vi "Outputs.vi"(8 "error in (no error)":errorcluster, 11 "State in":T1={"State"=enum."Idle", "Start Time"=timestamp(0 s since 1904-01-01), "Configuration"={"Cycle Period"=0.0, "Setpoint Entry"=0.0, "Output Device"=enum."Huber Ministat 230", "Huber Ministat 230 Settings"={"VISA resource name"="", "Simulated?"=FALSE}, "Lauda Settings"={"VISA resource name"="", "Simulated?"=FALSE, "Pump Power"=2}, "Julabo FP-50 Settings"={"VISA resource name"="", "Simulated?"=FALSE, "Pump Power"=2}, "Internal Control?"=FALSE, "Huber Unistat 410 Settings"={"VISA resource name"="", "Address"=0, "Simulated?"=FALSE}}, "Current Time"=timestamp(0 s since 1904-01-01), "First Iteration"=FALSE, "Data"={"TCU Speed"=0.0, "Temperature"=0.0}, "Process Name"="", "TCU On?"=FALSE, "Output Error"=FALSE, "Start Log"=FALSE, "Power Level Changed"=FALSE} {"Configuration"."Huber Unistat 410 Settings"."Address" min=0 max=99 format="%02.0f"; "Configuration"."Julabo FP-50 Settings"."Pump Power" min=0 max=8 step=1; "Configuration"."Lauda Settings"."Pump Power" min=0 max=8 step=1}) -> (0 "error out":errorcluster, 3 "State out":T1={"State"=enum."Idle", "Start Time"=timestamp(0 s since 1904-01-01), "Configuration"={"Cycle Period"=0.0, "Setpoint Entry"=0.0, "Output Device"=enum."Huber Ministat 230", "Huber Ministat 230 Settings"={"VISA resource name"="", "Simulated?"=FALSE}, "Lauda Settings"={"VISA resource name"="", "Simulated?"=FALSE, "Pump Power"=2}, "Julabo FP-50 Settings"={"VISA resource name"="", "Simulated?"=FALSE, "Pump Power"=2}, "Internal Control?"=FALSE, "Huber Unistat 410 Settings"={"VISA resource name"="", "Address"=0, "Simulated?"=FALSE}}, "Current Time"=timestamp(0 s since 1904-01-01), "First Iteration"=FALSE, "Data"={"TCU Speed"=0.0, "Temperature"=0.0}, "Process Name"="", "TCU On?"=FALSE, "Output Error"=FALSE, "Start Log"=FALSE, "Power Level Changed"=FALSE} {"Configuration"."Huber Unistat 410 Settings"."Address" min=0 max=99 format="%02.0f"; "Configuration"."Julabo FP-50 Settings"."Pump Power" min=0 max=8 step=1; "Configuration"."Lauda Settings"."Pump Power" min=0 max=8 step=1})   [LabVIEW 2018, in "TCU Module.lvlib" / "TCU Module Engine.lvlib"]
uses:
  TCU Module Engine.lvlib
  TCU State Cluster.ctl
  State Enum.ctl
  TCU Module Settings Cluster.ctl
  Output Devices.ctl
  Huber TCU/Huber Settings.ctl
  Lauda Integral XT-150 TCU/Lauda Settings.ctl
  Julabo Type 1 TCU/Julabo Type 1 TCU Folder/Julabo FP-50 Settings.ctl
  Huber Unistat 410 TCU/Huber Unistat 410 RS485 Settings.ctl
  Tag VIs/Tag FGV Operation Enum.ctl
  Shared Variables/Dynamic Shared Variables.lvlib
  Huber TCU/Huber Ministat 230 TCU.lvlib
  Lauda Integral XT-150 TCU/Lauda TCU.lvlib
  Julabo Type 1 TCU/Julabo Type 1 TCU Folder/Julabo Type FP-50 TCU.lvlib
  Huber Unistat 410 TCU/Huber Unistat 410 TCU.lvlib
  TCU Module.lvlib
panel:
  # "Output Instruments"
  # "Output Instruments"
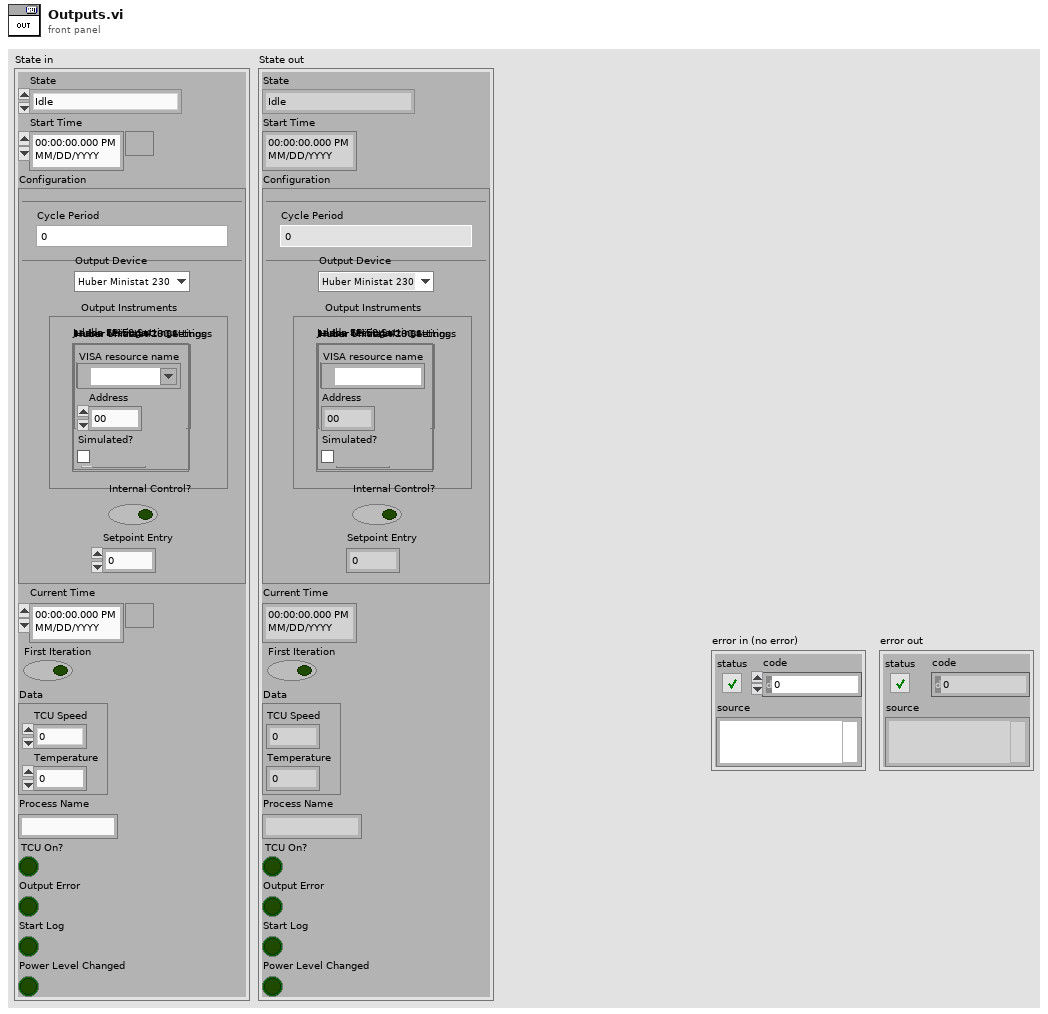
[diagram p1: front panel]
types:
  T1 = typedef "TCU Module.lvlib/TCU Module Engine.lvlib/TCU State Cluster.ctl" = cluster{"State":T2, "Start Time":timestamp, "Configuration":T3, "Current Time":timestamp, "First Iteration":bool, "Data":cluster{"TCU Speed":dbl, "Temperature":dbl}, "Process Name":string, "TCU On?":bool, "Output Error":bool, "Start Log":bool, "Power Level Changed":bool}
  T2 = typedef "TCU Module.lvlib/TCU Module Engine.lvlib/State Enum.ctl" = enum16{"Measuring", "Idle", "Paused"}
  T3 = typedef "TCU Module.lvlib/TCU Module Settings Cluster.ctl" = cluster{"Cycle Period":dbl, "Setpoint Entry":dbl, "Output Device":T4, "Huber Ministat 230 Settings":T5, "Lauda Settings":T6, "Julabo FP-50 Settings":T7, "Internal Control?":bool, "Huber Unistat 410 Settings":T8}
  T4 = typedef "Output Devices.ctl" = enum16{"Default", "Huber Ministat 230", "Huber Unistat 410", "Lauda XT-150", "Julabo FP-50"}
  T5 = typedef "Huber Ministat 230 TCU.lvlib/Huber Settings.ctl" = cluster{"VISA resource name":refnum<visa-resource-name>, "Simulated?":bool}
  T6 = typedef "Lauda TCU.lvlib/Lauda Settings.ctl" = cluster{"VISA resource name":refnum<visa-resource-name>, "Simulated?":bool, "Pump Power":i32}
  T7 = typedef "Julabo Type FP-50 TCU.lvlib/Julabo FP-50 Settings.ctl" = cluster{"VISA resource name":refnum<visa-resource-name>, "Simulated?":bool, "Pump Power":i32}
  T8 = typedef "Huber Unistat 410 TCU.lvlib/Huber Unistat 410 RS485 Settings.ctl" = cluster{"VISA resource name":refnum<visa-resource-name>, "Address":i8, "Simulated?":bool}
  T9 = typedef "Tag FGV Operation Enum.ctl" = enum16{"Init", "Set Notification Queue", "Create Tag", "Commit", "Write Tag (Numeric)", "Write Tag (Boolean)", "Read All Tags", "Read One Tag", "Delete Tag Category", "Set Alarm Parameters (Numeric)", "Set Alarm Parameters (Boolean)", "Enable All Alarms", "Disable All Alarms", "Delete All Tags", "Read Alarms", "Ack Alarm", "Read Alarm Parameters (Numeric)", "Read Alarm Parameters (Boolean)"}
  T10 = typedef "TCU Module.lvlib/TCU Module Tag Names Cluster.ctl" = cluster{"TCU Temp":string, "Output Device Tag":string, "TCU Speed":string, "Identifier Tag":string}
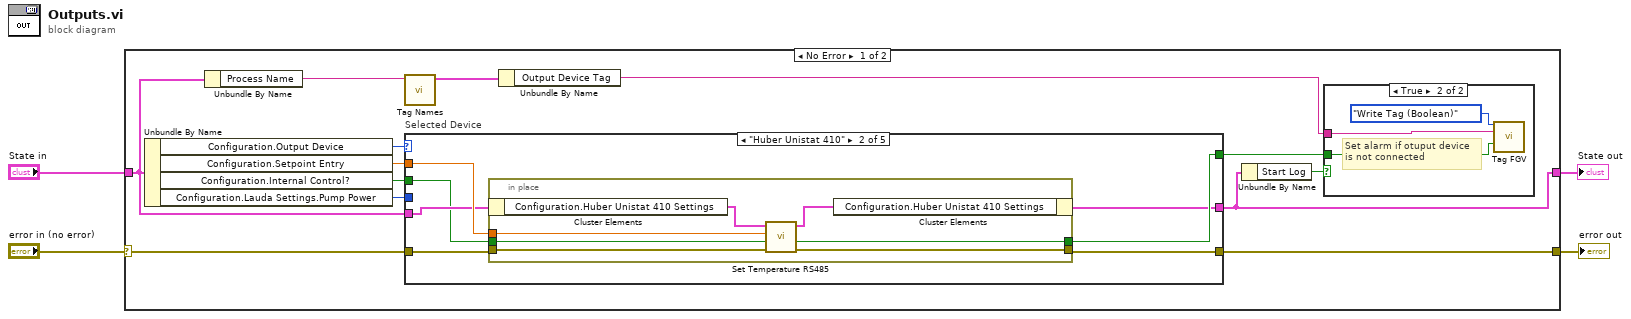
[diagram p0: block diagram]
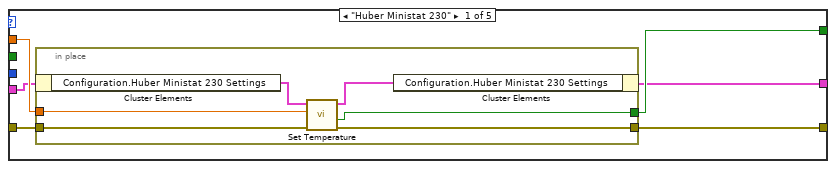
[diagram p3: hidden frame]
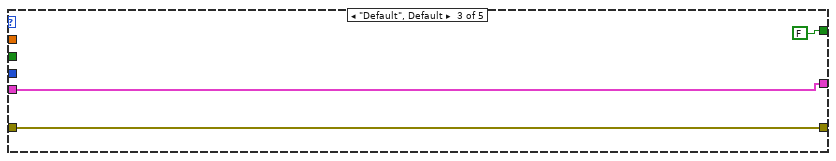
[diagram p4: hidden frame]
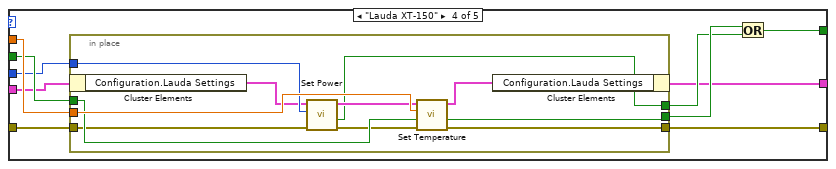
[diagram p5: hidden frame]
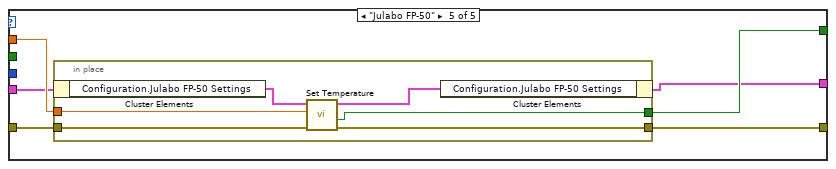
[diagram p6: hidden frame]
diagram:
  n1 = case shown="No Error" "error in (no error)" {
    selector: "error in (no error)" -> [w15 w84]
    tunnel: [w12 w84] -> w3
    tunnel: "State in" -> [w11 w83]
    tunnel: [w7 w83] -> w1
    frame No Error {
      n2 = Unbundle By Name(w11) -> ("Configuration.Output Device"=w17:T4, "Configuration.Setpoint Entry"=w16:dbl, "Configuration.Internal Control?"=w6:bool, "Configuration.Lauda Settings.Pump Power"=w5:i32)
      n3 = Unbundle By Name(w11) -> ("Process Name"=w14:string)
      n4 = call "Tag Names.vi"("Process Name"=w14) -> ("Pump Module Tag Names"=w13:T10)  [unwired: 8 in, 2 out]
      n5 = case "Selected Device" shown="\"Huber Unistat 410\"" w17 {
        tunnel: w16 -> [w23 w36 _ w59 w73]
        tunnel: w15 -> [w26 w39 w48 w56 w76]
        tunnel: [w25 w38 w48 w58 w75] -> w12
        tunnel: w11 -> [w22 w35 w49 w51 w72]
        tunnel: [w21 w34 w49 w50 w71] -> w7
        tunnel: [w24 w37 FALSE ("Connection Error") w52 w74] -> w9
        tunnel: w6 -> [_ w33 _ w57 _]
        tunnel: w5 -> [_ _ _ w55 _]
        frame "Huber Ministat 230" {
          n6 = in-place {
            in-place-border: w26 -> [w32]
            in-place-border: [w31] -> w25
            in-place-border: [w30] -> w24
            in-place-border: w23 -> [w29]
            n7 = in-place-cluster #1(w22) -> ("Configuration.Huber Ministat 230 Settings"=w28:T5)
            n8 = call "Set Temperature.vi"("error in (no error)"=w32, "Setpoint"=w29, "Huber Settings In"=w28) -> ("error out"=w31:errorcluster, "Connection Error"=w30:bool, "Huber Settings Out"=w27:T5)  [unwired: 6 in]
            n9 = in-place-cluster #1("Configuration.Huber Ministat 230 Settings"=w27) -> (w21:T1)
          }
        }
        frame "Huber Unistat 410" {
          n10 = in-place {
            in-place-border: w39 -> [w44]
            in-place-border: [w43] -> w38
            in-place-border: [w41] -> w37
            in-place-border: w36 -> [w45]
            in-place-border: w33 -> [w40]
            n11 = in-place-cluster #2(w35) -> ("Configuration.Huber Unistat 410 Settings"=w46:T8)
            n12 = call "Set Temperature RS485.vi"("error in (no error)"=w44, "Internal?"=w40, "Setpoint"=w45, "Huber Unistat 410 Settings"=w46) -> ("error out"=w43:errorcluster, "Connection Error"=w41:bool, "Huber Unistat 410 Settings"=w42:T8)  [unwired: 5 in]
            n13 = in-place-cluster #2("Configuration.Huber Unistat 410 Settings"=w42) -> (w34:T1)
          }
        }
        frame "Default", Default {
        }
        frame "Lauda XT-150" {
          n14 = in-place {
            in-place-border: w59 -> [w70]
            in-place-border: [w69] -> w58
            in-place-border: w57 -> [w68]
            in-place-border: w56 -> [w66]
            in-place-border: w55 -> [w64]
            in-place-border: [w63] -> w54
            in-place-border: [w62] -> w53
            n15 = in-place-cluster #3(w51) -> ("Configuration.Lauda Settings"=w60:T6)
            n16 = call "Set Power.vi"("error in (no error)"=w66, "Power"=w64, "Lauda Settings In"=w60) -> ("error out"=w65:errorcluster, "Connection Error"=w62:bool, "Lauda Settings Out"=w67:T6)  [unwired: 6 in]
            n17 = call "Set Temperature.vi"("error in (no error)"=w65, "Internal?"=w68, "Setpoint"=w70, "Lauda Settings In"=w67) -> ("error out"=w69:errorcluster, "Connection Error"=w63:bool, "Lauda Settings Out"=w61:T6)  [unwired: 5 in]
            n18 = in-place-cluster #3("Configuration.Lauda Settings"=w61) -> (w50:T1)
          }
          n19 = Or(x=w54, y=w53) -> (x .or. y?=w52:bool)
        }
        frame "Julabo FP-50" {
          n20 = in-place {
            in-place-border: w76 -> [w82]
            in-place-border: [w81] -> w75
            in-place-border: [w80] -> w74
            in-place-border: w73 -> [w79]
            n21 = in-place-cluster #4(w72) -> ("Configuration.Julabo FP-50 Settings"=w78:T7)
            n22 = call "Set Temperature.vi"("error in (no error)"=w82, "Setpoint"=w79, "Julabo Fp-50 Settings"=w78) -> ("error out"=w81:errorcluster, "Connection Error"=w80:bool, "Julabo FP-50 Settings"=w77:T7)  [unwired: 6 in]
            n23 = in-place-cluster #4("Configuration.Julabo FP-50 Settings"=w77) -> (w71:T1)
          }
        }
      }
      n24 = Unbundle By Name(w13) -> ("Output Device Tag"=w10:string)
      n25 = Unbundle By Name(w7) -> ("Start Log"=w8:bool)
      n26 = case shown="True" w8 {
        tunnel: w10 -> [_ w20]
        tunnel: w9 -> [_ w19]
        frame False {
        }
        frame True {
          # "Set alarm if otuput device\nis not connected"
          n27 = call "Tag FGV.vi"("Operation"=Tag_FGV_Operation_Enum."Write Tag (Boolean)", "Tag Name"=w20, "Data"=w19) -> ()  [unwired: 5 in, 8 out]
        }
      }
    }
    frame Error {
    }
  }
  "error out" <- w3
  "State out" <- w1
